vi "ex14-6(withSubVI).vi"() -> ()   [LabVIEW 2014]
panel:
  out "溢位?65536(減法)":bool
  out "溢位?65536(加法)":bool
  in  "X":dbl
  in  "Y":dbl
  in  "SUB":bool
  out "X-Y":dbl
  out "X+Y":dbl
  in  "ADD":bool
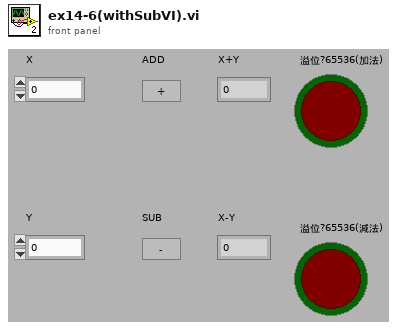
[diagram p1: front panel]
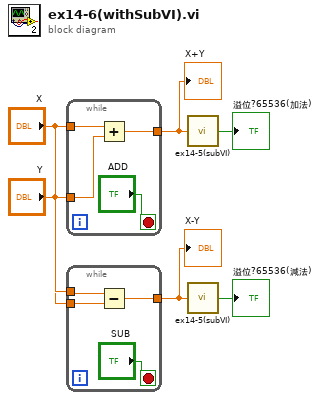
[diagram p0: block diagram]
diagram:
  n1 = while {
    tunnel: [w9] -> w3
    tunnel: "X" -> [w8]
    tunnel: "Y" -> [w7]
    stop <- "ADD" stop-if-true
    n2 = Add(x=w8, y=w7) -> (x+y=w9:dbl)
  }
  "X+Y" <- w3
  n3 = while {
    tunnel: [w13] -> w1
    tunnel: "X" -> [w12]
    tunnel: "Y" -> [w11]
    stop <- "SUB" stop-if-true
    n4 = Subtract(x=w12, y=w11) -> (x-y=w13:dbl)
  }
  "X-Y" <- w1
  n5 = call "ex14-5(subVI).vi"("輸入"=w3) -> ("溢位?65536"=→"溢位?65536(加法)":bool)
  n6 = call "ex14-5(subVI).vi"("輸入"=w1) -> ("溢位?65536"=→"溢位?65536(減法)":bool)
